vi "Get_users_email_addresses.vi"(1 "OK":bool) -> ()   [LabVIEW 2022 SP3]
uses:
  File/Setup_Filetype.ctl
  Globals/Meas_global.vi
  Globals/Preference_global.vi
panel:
  out "Times Mon - Fri":string[](array[string])=["Midnight to 1am", "1am to 2am", "2am to 3am", "3am to 4am", "4am to 5am", "5am to 6am", "6am to 7am", "7am to 8am", "8am to 9am", "9am to 10am", "10am to 11am", "11am to Midday", "Midday to 1pm", "1pm to 2pm", "2pm to 3pm", "3pm to 4pm", "4pm to 5pm", "5pm to 6pm", "6pm to 7pm", "7pm to 8pm", "8pm to 9pm", "9pm to 10pm", "10pm to 11pm", "11pm to Midnight"]
  out "Message":string
  in  "Email addresses":string[](array[string])
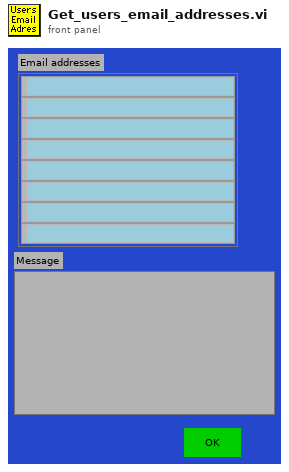
[diagram p1: front panel]
types:
  T1 = typedef "Setup_Filetype.ctl" = enum16{"Measurement Setups", "Calibration Setups", "General", "Results File Plotter Setups", "Speed Calib Tweaks"}
  T2 = enum16{"Highest", "High", "Normal", "Low", "Lowest"}
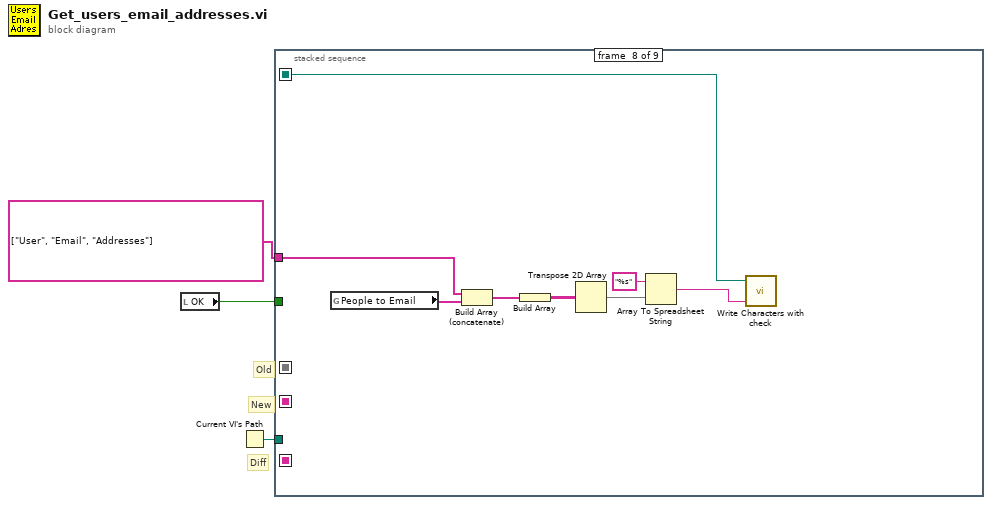
[diagram p0: block diagram]
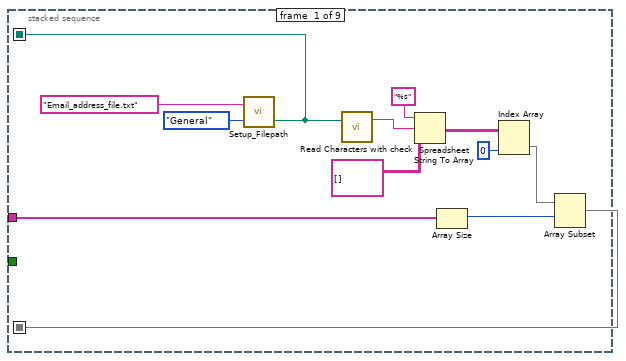
[diagram p2: hidden frame]
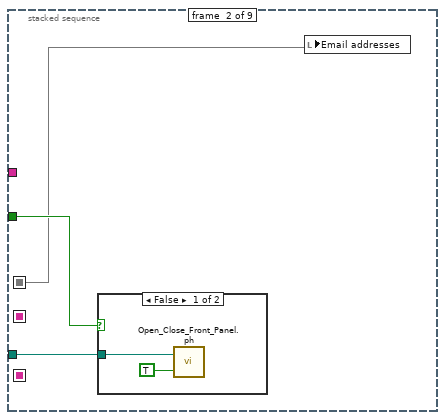
[diagram p3: hidden frame]
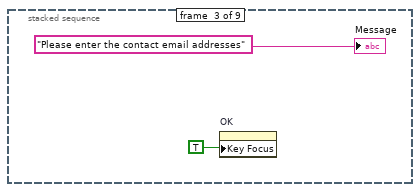
[diagram p5: hidden frame]
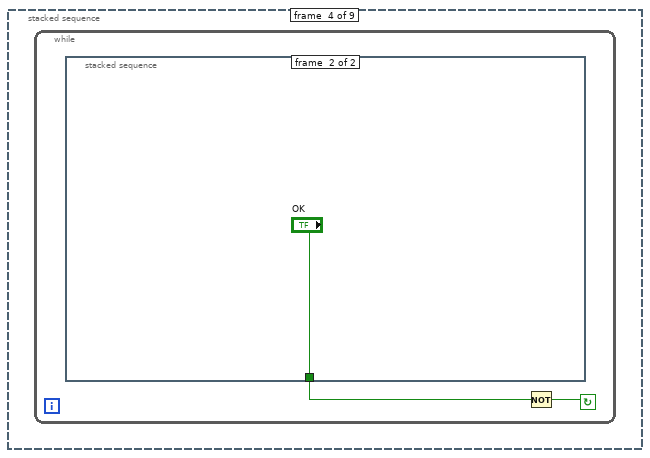
[diagram p6: hidden frame]
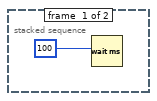
[diagram p7: hidden frame]
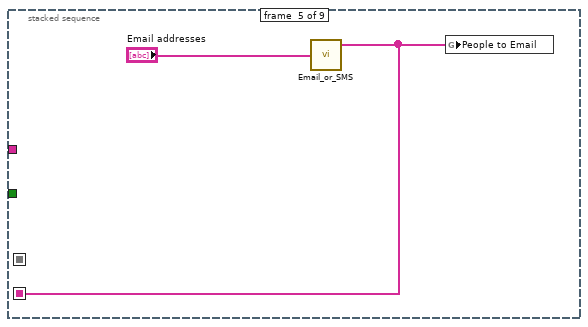
[diagram p8: hidden frame]
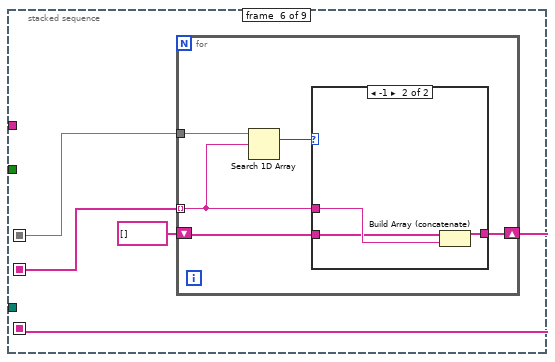
[diagram p9: hidden frame]
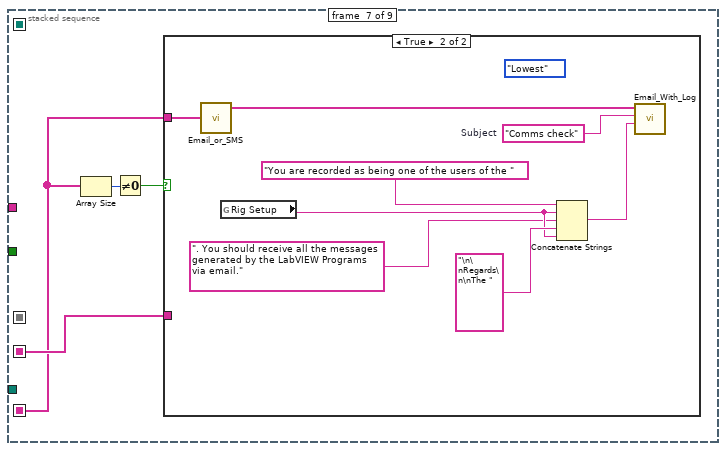
[diagram p11: hidden frame]
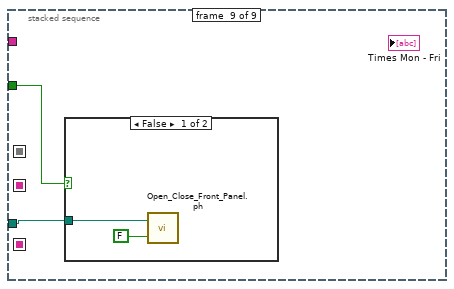
[diagram p13: hidden frame]
diagram:
  # "Diff"
  # "Old"
  # "New"
  n1 = local read "OK"() -> (w2:bool)
  n2 = Current VI's Path() -> (path=w3:path)
  n3 = stacked-sequence {
    seq-local: [_ _ _ _ w27 _ _ _ _] -> [_ _ _ _ _ w29 w44 _ _]
    seq-local: [w5 _ _ _ _ _ _ _ _] -> [_ _ _ _ _ _ _ w55 _]
    seq-local: [w6 _ _ _ _ _ _ _ _] -> [_ w16 _ _ _ w32 _ _ _]
    seq-local: [_ _ _ _ _ w30 _ _ _] -> [_ _ _ _ _ _ w43 _ _]
    tunnel: w3 -> [_ w18 _ _ _ _ _ _ w63]
    tunnel: w2 -> [_ w17 _ _ _ _ _ _ w62]
    tunnel: string[] ["User", "Email", "Addresses"] ("array") -> [w9 _ _ _ _ _ _ w58 _]
    frame #0 {
      n4 = call "Setup_Filepath.vi"("Setup File Type"=Setup_Filetype."General", "Filename in"="Email_address_file.txt" ("Substring")) -> ("Filename Out"=w5:path)  [unwired: 1 out]
      n5 = call "Read Characters with check.vi"("file (use dialog)"=w5) -> ("Read String"=w4:string)  [unwired: 1 in, 1 out]
      n6 = Spreadsheet String To Array(format string="%s", spreadsheet string=w4, array type (2D Dbl)=string[][] []) -> (array=w10:string[][])  [unwired: 1 in]
      n7 = Array Size(array=w9) -> (size(s)=w7:i32)
      n8 = Index Array(array=w10, index (col)=0 ("disabled index (col)")) -> (element=w8:string[])  [unwired: 1 in]
      n9 = Array Subset(array=w8, index=w7) -> (w6:string[])  [unwired: 1 in]
    }
    frame #1 {
      n10 = case shown="False" w17 {
        tunnel: w18 -> [w20 _]
        frame False {
          n11 = call "Open_Close_Front_Panel.ph.vi"("openWindow (T)"=TRUE ("Front Panel Window:Open"), "VI path"=w20) -> ()  [unwired: 1 in, 1 out]
        }
        frame True {
        }
      }
      n12 = local write "Email addresses"(w16) -> ()
    }
    frame #2 {
      n13 = property on="OK" class="Bool (strict)"("Key Focus"=TRUE ("Write Attribute")) -> ()  [unwired: 2 in, 2 out]
      "Message" <- "Please enter the contact email addresses" ("Message")
    }
    frame #3 {
      n14 = while {
        stop <- w24 continue-if-true
        n15 = stacked-sequence {
          tunnel: [_ "OK"] -> w23
          frame #0 {
            n16 = Wait (ms)(milliseconds to wait=u32 100 ("milliseconds to Wait")) -> ()  [unwired: 1 out]
          }
          frame #1 {
          }
        }
        n17 = Not(x=w23) -> (.not. x?=w24:bool)
      }
    }
    frame #4 {
      n18 = call "Email_or_SMS.vi"("Email address"="Email addresses") -> ("Email"=w27:string[])  [unwired: 3 out]
      n19 = global write "Meas_global.vi" "People to Email"(w27) -> ()
    }
    frame #5 {
      n20 = for {
        tunnel: w32 -> [w37]
        shift-right: [w34] -> w30
        shift-left: string[] [] -> [w35]
        tunnel: w29 -> [w33] mode=indexing
        n21 = Search 1D Array(1D array=w37, element=w33) -> (index of element=w36:i32)  [unwired: 1 out]
        n22 = case shown="-1" w36 {
          tunnel: w33 -> [_ w41]
          tunnel: w35 -> [w38 w40]
          tunnel: [w38 w39] -> w34
          frame 0, Default {
          }
          frame -1 {
            n23 = Build Array (concatenate)(w40, w41) -> (w39:string[])
          }
        }
      }
    }
    frame #6 {
      n24 = Array Size(array=w43) -> (size(s)=w45:i32)
      n25 = Not Equal To 0?(x=w45) -> (x != 0?=w42:bool)
      n26 = case shown="True" w42 {
        tunnel: w43 -> [_ w51]
        tunnel: w44 -> [_ _]
        frame False {
        }
        frame True {
          (unwired) T2."Lowest" ("Priorities")
          w47 = "Comms check"  # Subject
          n27 = call "Email_or_SMS.vi"("Email address"=w51) -> ("Email"=w50:string[])  [unwired: 3 out]
          n28 = global read "Preference_global.vi" "Rig Setup"() -> (w49:string)
          n29 = Concatenate Strings("You are recorded as being one of the users of the " ("Message"), w49, ". You should receive all the messages generated by the LabVIEW Programs via email." ("Message"), "\n\nRegards\n\nThe " ("Message"), w49) -> (w48:string)
          n30 = call "Email_With_Log.vi"("recipients"=w50, "subject ([No Subject])"=w47, "message"=w48) -> ()  [unwired: 1 in, 3 out]
        }
      }
    }
    frame #7 {
      n31 = global read "Meas_global.vi" "People to Email"() -> (w61:string[])
      n32 = Build Array (concatenate)(w58, w61) -> (w57:string[])
      n33 = Build Array(w57) -> (w56:string[][])
      n34 = Transpose 2D Array(2D array=w56) -> (transposed array=w60:string[][])
      n35 = Array To Spreadsheet String(array=w60, 3:"%s" ("format string")) -> (spreadsheet string=w54:string)  [unwired: 1 in]
      n36 = call "Write Characters with check.vi"("String to Write"=w54, "file (use dialog)"=w55) -> ()  [unwired: 2 in, 1 out]
    }
    frame #8 {
      n37 = case shown="False" w62 {
        tunnel: w63 -> [w64 _]
        frame False {
          n38 = call "Open_Close_Front_Panel.ph.vi"("openWindow (T)"=FALSE ("Front Panel Window:Open"), "VI path"=w64) -> ()  [unwired: 1 in, 1 out]
        }
        frame True {
        }
      }
    }
  }
